vi "Get Byte Count Field Width.vi"(8 "error in (no error)":errorcluster, 11 "RFFE Extended Command in":refnum<class "RFFE Extended Command.lvclass">) -> (0 "error out":errorcluster, 2 "Byte Count Field Width":i32, 3 "RFFE Extended Command out":refnum<class "RFFE Extended Command.lvclass">)   [LabVIEW 2018, in "MIPI RFFE API.lvlib" / "RFFE Extended Command.lvclass"]
uses:
  RFFE Extended Command.lvclass
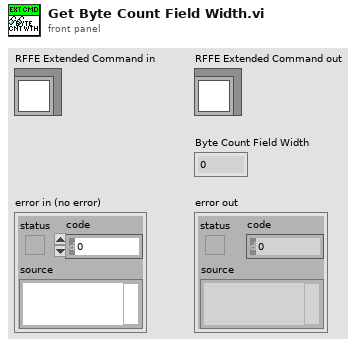
[diagram p1: front panel]
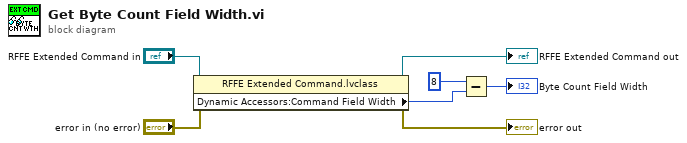
[diagram p0: block diagram]
diagram:
  n1 = property class="RFFE Extended Command.lvclass"(reference="RFFE Extended Command in", error in="error in (no error)") -> (reference out=→"RFFE Extended Command out":refnum<class "RFFE Extended Command.lvclass">, error out=→"error out":errorcluster, "Dynamic Accessors:Command Field Width"=w1:i32)
  n2 = Subtract(x=8 ("y"), y=w1) -> (x-y=→"Byte Count Field Width":i32)
